vi "MH_T2 Read Acq QueueClassic.vi"() -> ()   [LabVIEW 2019]
uses:
  <userlib>/MultiHarp150/T2Lib/MH_T2QMessage.ctl
  <userlib>/MultiHarp150/T2Lib/MH_T2DeltaQMessage.ctl
panel:
  in  "Dbuffsize":i32=10
  out "Done":bool
  out "TotalRec":i32
  out "TotalTime":u32
  in  "stop":bool
  out "sortie d'erreur":errorcluster caption="ErrorOut"
  out "RollOver":bool
  in  "BufSze":i32=1000000
  in  "entrée d'erreur":errorcluster caption="ErrorIn"
  in  "WIndowW":i32
  in  "Save Data":bool
  in  "Correl Ch":u32=2
  in  "Base Ch":u32=1
  in  "refnum":refnum<file>
  out "DeltaT":u32[](array[numeric])
  out "nActual":i32[](array[numeric])
  out "En Attente":i32[](array[numeric])
  out "Tableau":u64[][](array[numeric])
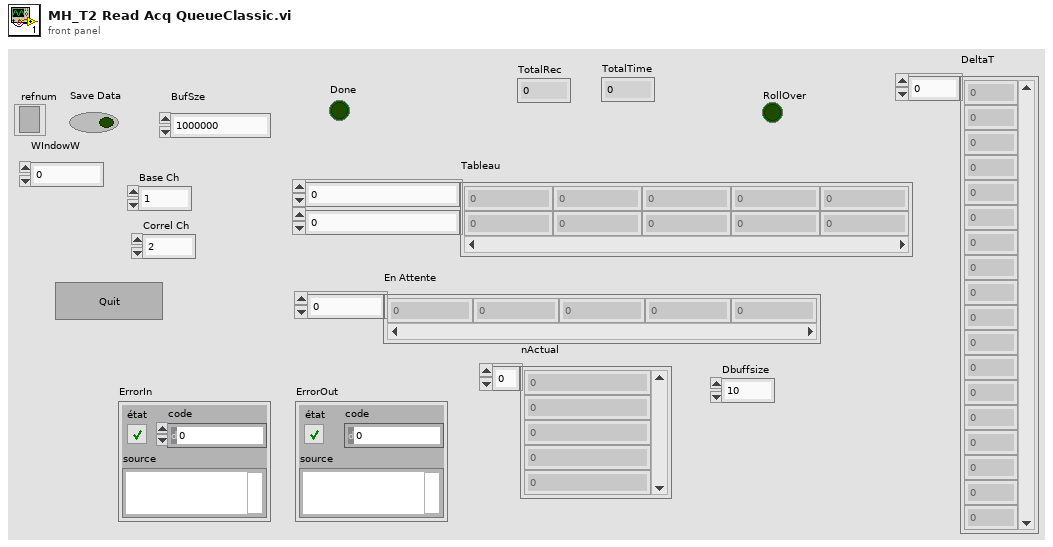
[diagram p1: front panel]
types:
  T1 = typedef "MH_T2DeltaQMessage.ctl" = cluster{"Message":string, "buffer":i32[], "Code":i32, "nactual":i32}
  T2 = typedef "MH_T2QMessage.ctl" = cluster{"Message":string, "buffer":u32[], "Code":i32, "nactual":i32}
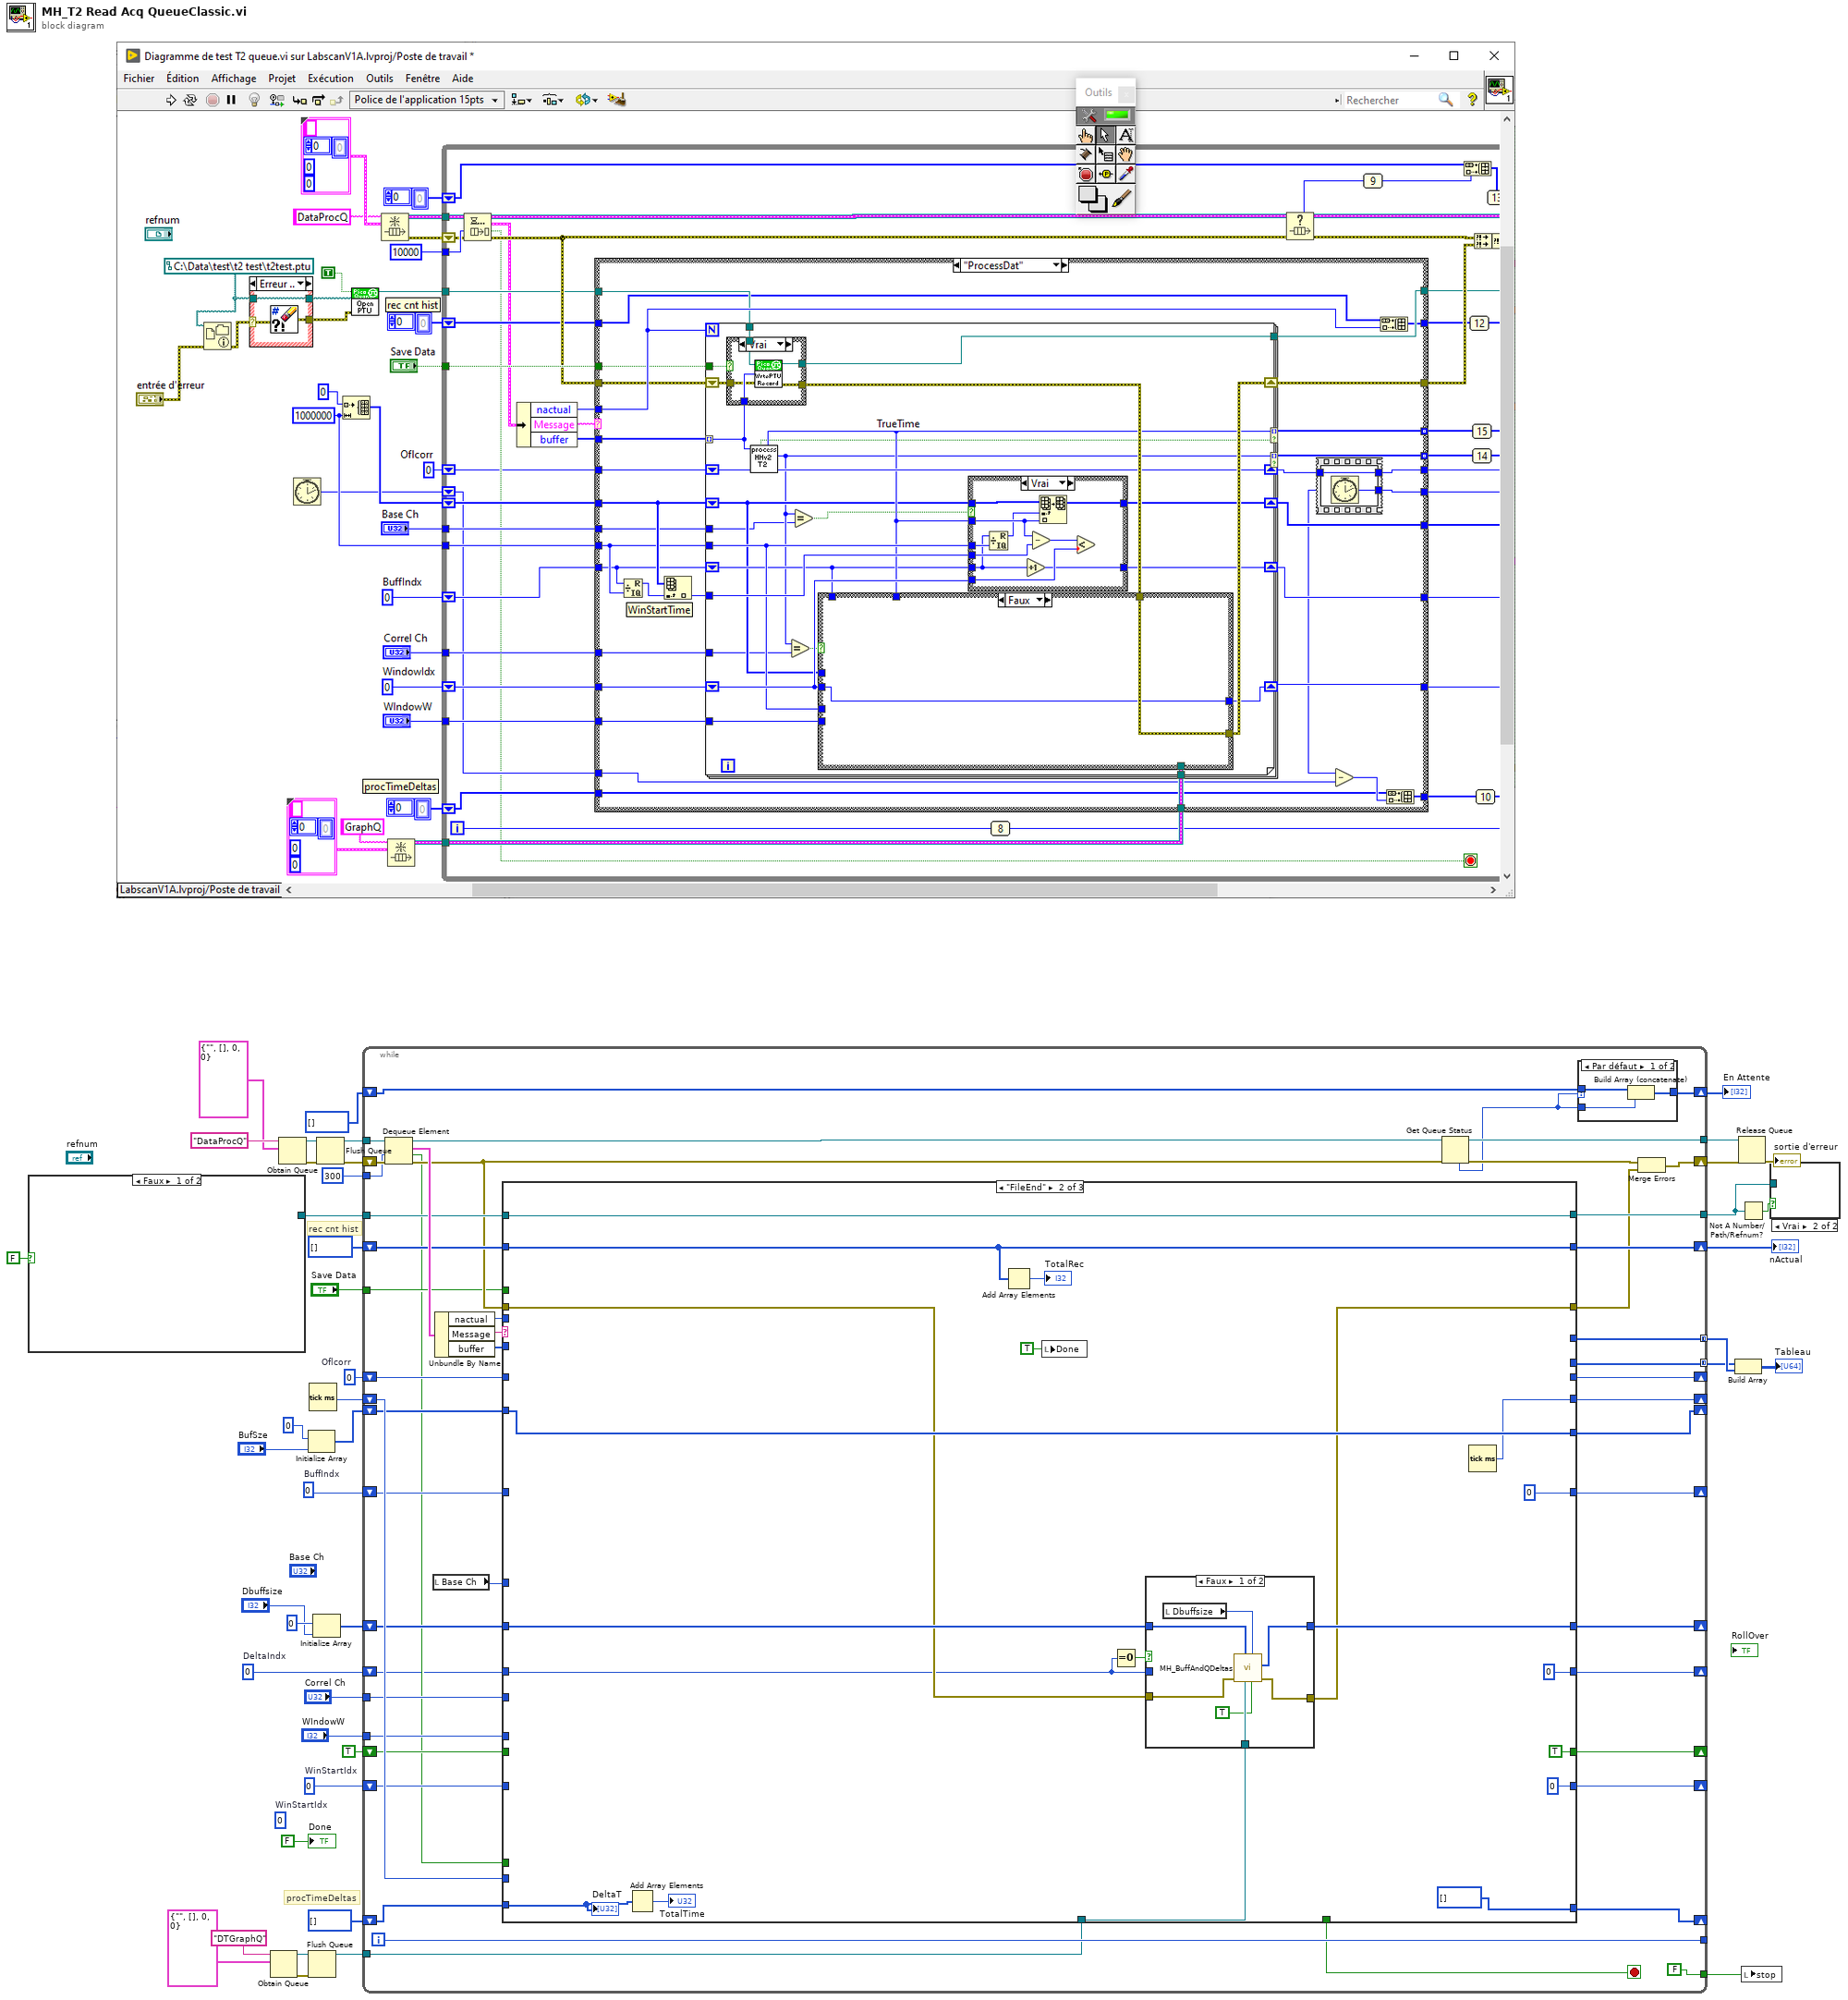
[diagram p0: block diagram]
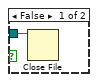
[diagram p2: hidden frame]
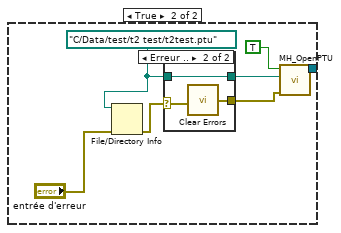
[diagram p3: hidden frame]
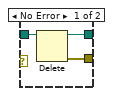
[diagram p4: hidden frame]
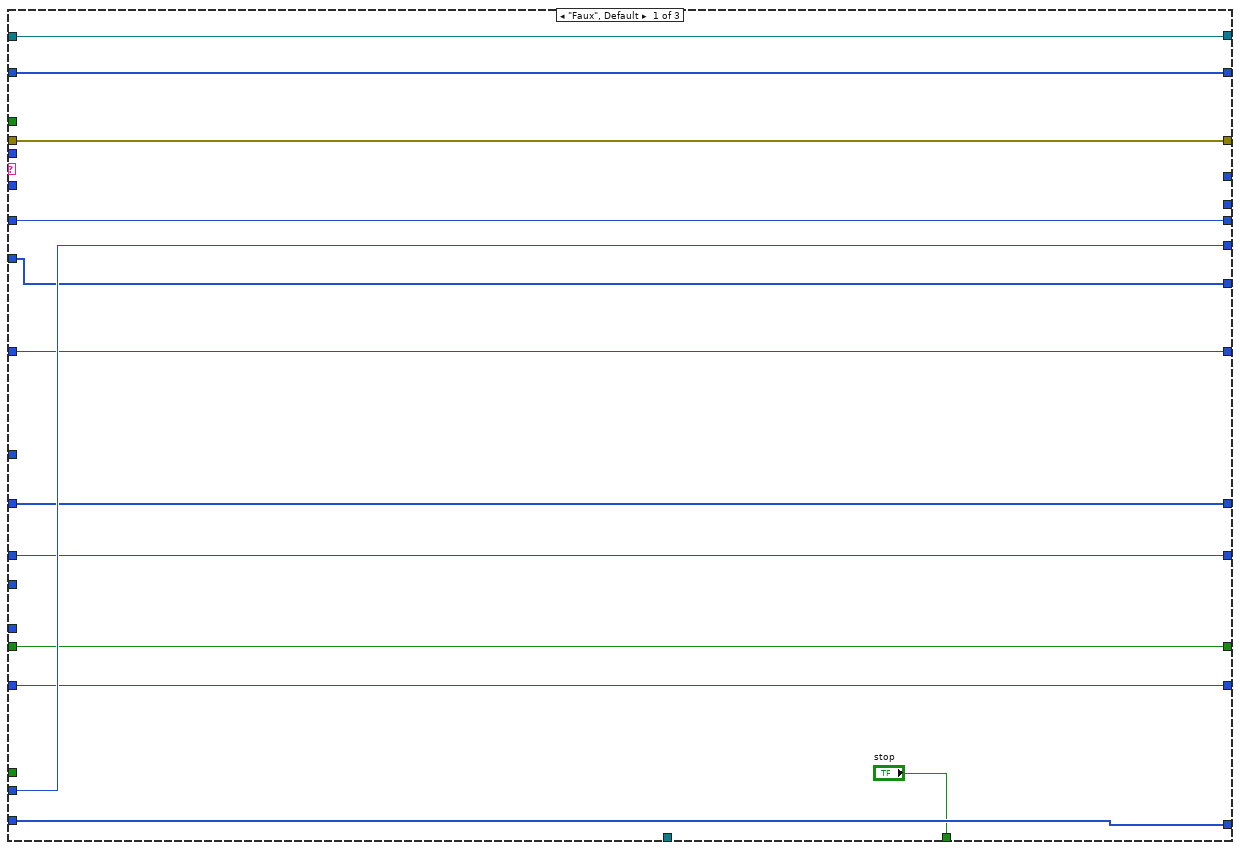
[diagram p6: hidden frame]
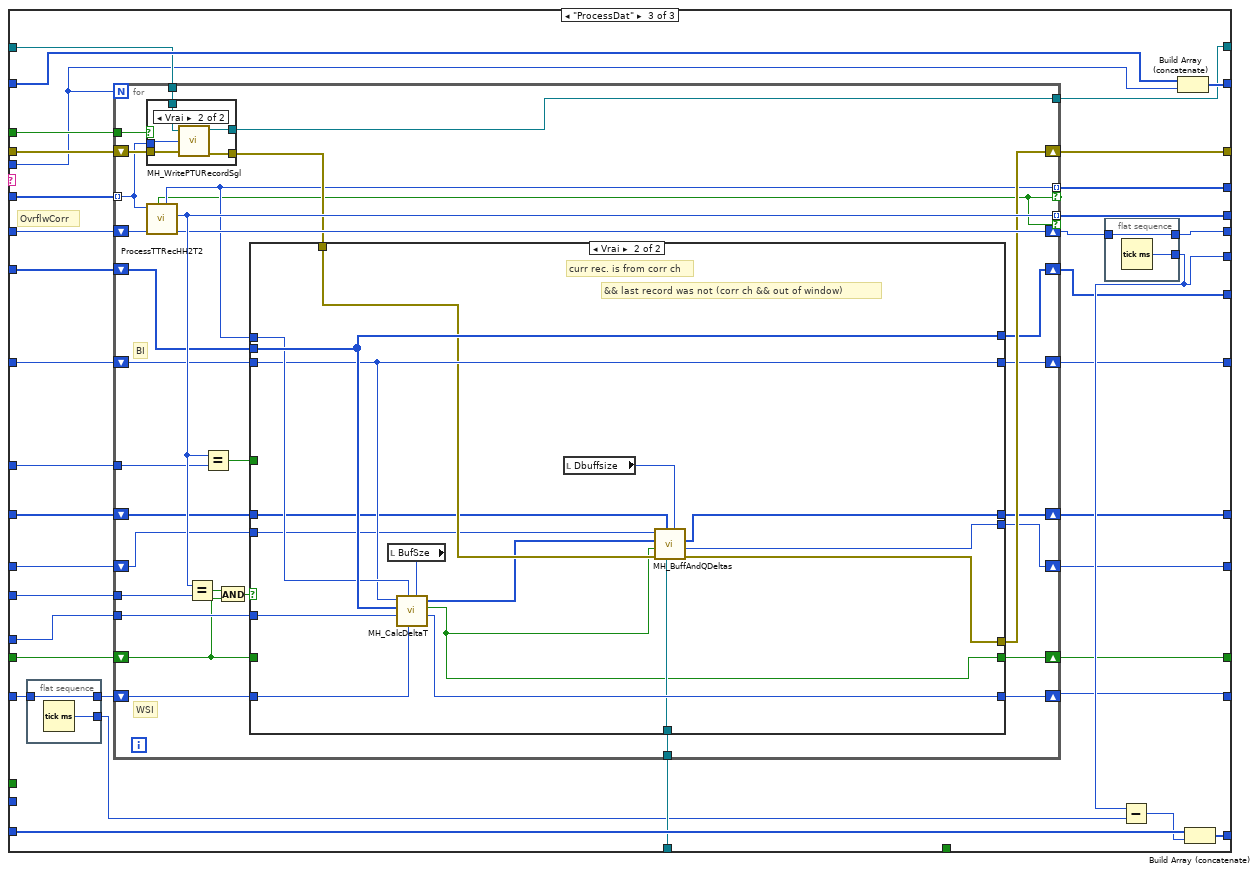
[diagram p8: hidden frame]
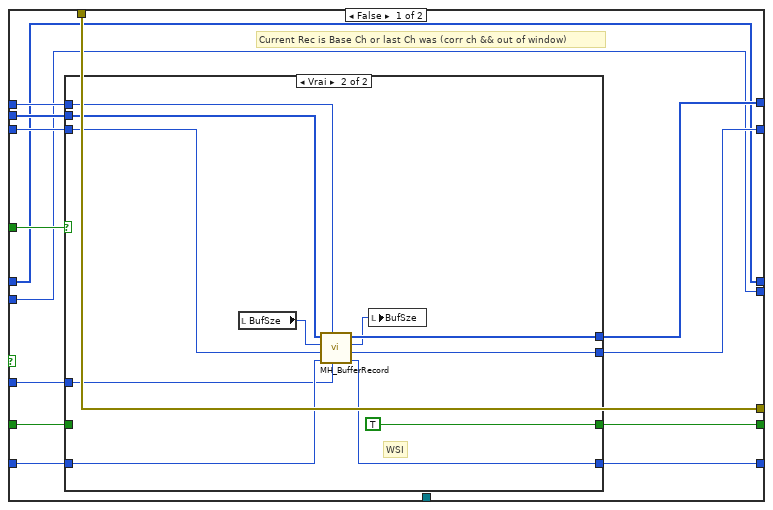
[diagram p10: hidden frame]
diagram:
  (unwired) 0  # WinStartIdx
  w3 = 0  # DeltaIndx
  w26 = 0  # WinStartIdx
  w14 = 0  # BuffIndx
  w42 = u64 0  # Oflcorr
  # "procTimeDeltas"
  # "rec cnt hist"
  n1 = case shown="Faux" FALSE {
    tunnel: [_ w50] -> w30
    frame False {
    }
    frame True {
      w47 = path "C:/Data/test/t2 test/t2test.ptu" ("chemin sélectionné")
      n2 = File/Directory Info(path=w47, error in="entrée d'erreur") -> (error out=w46:errorcluster)  [unwired: 6 out]
      n3 = case shown="Erreur .." w46 {
        selector: w46 -> [_ w56]
        tunnel: w47 -> [w54 w57]
        tunnel: [w53 w57] -> w49
        tunnel: [w52 w55] -> w48
        frame No Error {
          n4 = Delete(path (use dialog)=w54) -> (deleted path=w53:path, error out=w52:errorcluster)  [unwired: 4 in, 1 out]
        }
        frame Error {
          n5 = call <vilib>:"Clear Errors.vi"("error in (no error)"=w56) -> ("error out"=w55:errorcluster)  [unwired: 5 in, 1 out]
        }
      }
      n6 = call <userlib>:"MH_OpenPTU.vi"("ErrorIn"=w48, "chemin sélectionné"=w49, "WriteMode"=TRUE) -> ("refnum en sortie"=w50:refnum<file>)  [unwired: 6 in, 2 out]
    }
  }
  n7 = Obtain Queue(name (unnamed)="DTGraphQ" ("nom (aucun)"), element data type=T1 {"Message"="", "buffer"=[], "Code"=0, "nactual"=0} ("ClassQueue")) -> (queue out=w5:refnum<queue>, error out=w6:errorcluster)  [unwired: 3 in, 1 out]
  n8 = Obtain Queue(name (unnamed)="DataProcQ" ("nom (aucun)"), element data type=T2 {"Message"="", "buffer"=[], "Code"=0, "nactual"=0} ("ClassQueue")) -> (queue out=w11:refnum<queue>, error out=w8:errorcluster)  [unwired: 3 in, 1 out]
  n9 = Initialize Array(u64 0 ("truetime"), "BufSze") -> (w1:u64[])
  n10 = Flush Queue(queue=w5, error in (no error)=w6) -> (queue out=w16:refnum<queue>)  [unwired: 2 out]
  n11 = Tick Count (ms)() -> (millisecond timer value=w35:u32)
  n12 = Initialize Array(0 ("truetime"), "Dbuffsize") -> (w12:i32[])
  n13 = Flush Queue(queue=w11, error in (no error)=w8) -> (queue out=w10:refnum<queue>, error out=w9:errorcluster)  [unwired: 1 out]
  n14 = while {
    tunnel: w10 -> [w105]
    shift-right: [w83] -> w41
    shift-left: w9 -> [w106]
    shift-right: [w103] -> _
    shift-left: w42 -> [w104]
    tunnel: [w102] -> w38 mode=concatenating
    tunnel: [w99] -> _
    tunnel: [w95] -> w40
    tunnel: [w94] -> w37 mode=concatenating
    shift-right: [w92] -> _
    shift-left: w35 -> [w93]
    shift-right: [w90] -> _
    shift-left: u32[] [] ("DeltaT") -> [w91]
    shift-right: [w88] -> w32
    shift-left: i32[] [] ("DeltaT") -> [w89]
    shift-right: [w87] -> w39
    shift-left: i32[] [] ("DeltaT") -> [w86]
    tunnel: w30 -> [w85]
    tunnel: [w82] -> w19
    tunnel: "Save Data" -> [w81]
    shift-right: [w76] -> _
    shift-left: w1 -> [w80]
    shift-right: [w78] -> _
    shift-left: w14 -> [w79]
    tunnel: "Correl Ch" -> [w77]
    shift-right: [w72] -> _
    shift-left: w26 -> [w75]
    tunnel: "WIndowW" -> [w74]
    tunnel: 300 ("timeout en ms (-1)") -> [w73]
    tunnel: w16 -> [w70]
    shift-right: [w68] -> _
    shift-left: TRUE -> [w67]
    shift-right: [w65] -> _
    shift-left: w12 -> [w66]
    tunnel: [FALSE] -> w4
    shift-right: [w59] -> _
    shift-left: w3 -> [w60]
    i -> [w99]
    stop <- w63 stop-if-true
    n15 = Dequeue Element(queue=w105, timeout in ms (-1)=w73, error in (no error)=w106) -> (queue out=w97:refnum<queue>, element=w101:T2, timed out?=w64:bool, error out=w84:errorcluster)
    n16 = local read "Base Ch"() -> (w58:u32)
    n17 = Unbundle By Name(w101) -> ("nactual"=w71:i32, "Message"=w98:string, "buffer"=w100:u32[])
    n18 = case shown="\"FileEnd\"" w98 {
      tunnel: w104 -> [w123 _ w188]
      tunnel: [w123 _ w185] -> w103
      tunnel: [_ _ w187] -> w102
      tunnel: w100 -> [_ _ w178]
      tunnel: [_ _ w186] -> w94
      tunnel: w93 -> [w122 _ _]
      tunnel: [w121 u32[] [] ("DeltaT") w182] -> w90
      tunnel: [w122 w141 w179] -> w92
      tunnel: w91 -> [w121 w139 w184]
      tunnel: w89 -> [w120 w136 w181]
      tunnel: [w120 w136 w180] -> w88
      tunnel: w85 -> [w119 w143 w177]
      tunnel: w84 -> [w115 w127 w176]
      tunnel: [w119 w143 w175] -> w82
      tunnel: w81 -> [_ _ w174]
      tunnel: w80 -> [w117 w142 w163]
      tunnel: w79 -> [w118 _ w164]
      tunnel: [w118 0 ("BuffIndx") w172] -> w78
      tunnel: w77 -> [_ _ w173]
      tunnel: [w117 w142 w171] -> w76
      tunnel: w75 -> [w116 _ w157]
      tunnel: w74 -> [_ _ w170]
      tunnel: [w116 0 ("WinStartIdx") w168] -> w72
      tunnel: w71 -> [_ _ w167]
      tunnel: w70 -> [_ w126 w166]
      tunnel: [w115 w128 w165] -> w69
      tunnel: [w114 TRUE w162] -> w68
      tunnel: w67 -> [w114 _ w161]
      tunnel: w66 -> [w113 w130 w160]
      tunnel: [w113 w129 w159] -> w65
      tunnel: w64 -> [_ _ _]
      tunnel: ["stop" _ _] -> w63
      tunnel: w60 -> [w111 w125 w155]
      tunnel: [w111 0 w154] -> w59
      tunnel: w58 -> [_ _ w153]
      frame "Faux", Default {
      }
      frame "FileEnd" {
        n19 = Add Array Elements(numeric array=w139) -> (sum=→"TotalTime":u32)
        n20 = Add Array Elements(numeric array=w136) -> (sum=→"TotalRec":i32)
        n21 = local write "Done"(TRUE ("Done")) -> ()
        n22 = Equal To 0?(x=w125) -> (x = 0?=w124:bool)
        n23 = case shown="Faux" w124 {
          tunnel: w130 -> [w146 w152]
          tunnel: [w150 w152] -> w129
          tunnel: [w149 w151] -> w128
          tunnel: w127 -> [w148 w151]
          tunnel: w125 -> [_ _]
          tunnel: w126 -> [w147 _]
          frame False {
            n24 = local read "Dbuffsize"() -> (w145:i32)
            n25 = call <userlib>:"MH_BuffAndQDeltas.vi"("Force Write"=TRUE ("NewDelta"), "DBuffSize"=w145, "queue out"=w147, "DeltasBuffer"=w146, "erroIn"=w148) -> ("error out"=w149:errorcluster, "DeltasBufferOut"=w150:i32[])  [unwired: 4 in, 1 out]
          }
          frame True {
          }
        }
        n26 = Tick Count (ms)() -> (millisecond timer value=w141:u32)
        "DeltaT" <- w139
      }
      frame "ProcessDat" {
        # "OvrflwCorr"
        n27 = flat-sequence {
          tunnel: [w190] -> w156
          tunnel: w157 -> [w190]
          tunnel: [w189] -> w158
          frame #0 {
            n28 = Tick Count (ms)() -> (millisecond timer value=w189:u32)
          }
        }
        n29 = for {
          N: w167 -> [_]
          tunnel: [w205] -> w187 mode=indexing if=w196
          tunnel: w178 -> [w219] mode=indexing
          tunnel: [w217] -> w186 mode=indexing if=w196
          tunnel: w177 -> [w222]
          tunnel: [w220] -> w175
          tunnel: w174 -> [w218]
          shift-right: [w202] -> w171
          shift-left: w163 -> [w206]
          shift-right: [w203] -> w172
          shift-left: w164 -> [w204]
          tunnel: w173 -> [w215]
          tunnel: w170 -> [w214]
          shift-right: [w213] -> w169
          shift-left: w188 -> [w223]
          shift-right: [w212] -> w168
          shift-left: w156 -> [w208]
          shift-right: [w209] -> w165
          shift-left: w176 -> [w221]
          tunnel: w166 -> [w211]
          shift-right: [w201] -> w162
          shift-left: w161 -> [w199]
          shift-right: [w197] -> w159
          shift-left: w160 -> [w198]
          shift-right: [w194] -> w154
          shift-left: w155 -> [w195]
          tunnel: w153 -> [w193]
          # "BI"
          # "WSI"
          n30 = case shown="Vrai" w218 {
            tunnel: w222 -> [w224 w230]
            tunnel: w221 -> [w225 w229]
            tunnel: [w224 w228] -> w220
            tunnel: [w225 w227] -> w210
            tunnel: w219 -> [_ w226]
            frame False {
            }
            frame True {
              n31 = call <userlib>:"MH_WritePTURecordSgl.vi"("refnum"=w230, "TTTR Records"=w226, "error in"=w229) -> ("refnum en sortie"=w228:refnum<file>, "error out"=w227:errorcluster)  [unwired: 6 in]
            }
          }
          n32 = call <userlib>:"ProcessTTRecHH2T2.vi"("oflcorr_in"=w223, "rawbits"=w219) -> ("oflcorr_out"=w213:u64, "channel"=w217:u32, "truetime"=w205:u64, "is_photon"=w196:bool)  [unwired: 4 in, 2 out]
          n33 = Equal?(x=w217, y=w215) -> (x = y?=w216:bool)
          n34 = Equal?(x=w217, y=w193) -> (x = y?=w207:bool)
          n35 = And(x=w216, y=w199) -> (x .and. y?=w200:bool)
          n36 = case shown="Vrai" w200 {
            tunnel: w206 -> [w242 w276]
            tunnel: w208 -> [w238 w271]
            tunnel: w204 -> [w240 w273]
            tunnel: w214 -> [w236 w272]
            tunnel: [w235 w270] -> w212
            tunnel: w211 -> [_ w266]
            tunnel: w210 -> [w244 w269]
            tunnel: [w244 w265] -> w209
            tunnel: w207 -> [w241 _]
            tunnel: w205 -> [w237 w275]
            tunnel: [w239 w273] -> w203
            tunnel: [w243 w276] -> w202
            tunnel: [w234 w263] -> w201
            tunnel: w199 -> [w233 _]
            tunnel: w198 -> [w232 w262]
            tunnel: [w232 w268] -> w197
            tunnel: w195 -> [w231 w261]
            tunnel: [w231 w267] -> w194
            frame False {
              # "Current Rec is Base Ch or last Ch was (corr ch && out of window)"
              n37 = case shown="Vrai" w241 {
                tunnel: w242 -> [w247 w251]
                tunnel: w237 -> [_ w250]
                tunnel: w240 -> [w248 w254]
                tunnel: [w248 w258] -> w239
                tunnel: [w247 w257] -> w243
                tunnel: w238 -> [w246 w255]
                tunnel: w236 -> [_ w249]
                tunnel: [w246 w256] -> w235
                tunnel: [w245 TRUE] -> w234
                tunnel: w233 -> [w245 _]
                frame False {
                  # "could be sync or non-relevant channel"
                }
                frame True {
                  # "WSI"
                  n38 = local read "BufSze"() -> (w253:i32)
                  n39 = call <userlib>:"MH_BufferRecord.vi"("WindowWidth"=w249, "truetime"=w250, "WinIndex"=w255, "Buffindex"=w254, "Buffsize"=w253, "Buffer"=w251) -> ("WinIndexOut"=w256:i32, "BuffIndexOut"=w258:i32, "NewBuffsize"=w252:i32, "tableau (n rotations)"=w257:u64[])  [unwired: 2 in]
                  n40 = local write "BufSze"(w252) -> ()
                }
              }
            }
            frame True {
              # "&& last record was not (corr ch && out of window)"
              # "curr rec. is from corr ch"
              n41 = local read "BufSze"() -> (w274:i32)
              n42 = call <userlib>:"MH_CalcDeltaT.vi"("Buffsize"=w274, "WinIndex"=w271, "TrueTime"=w275, "WIndowW"=w272, "Data In"=w276, "Buffindex"=w273) -> ("WinIndexOut"=w270:i32, "NewDelta"=w263:bool, "DeltaT Out"=w260:i32[])  [unwired: 3 in]
              n43 = local read "Dbuffsize"() -> (w264:i32)
              n44 = call <userlib>:"MH_BuffAndQDeltas.vi"("DBuffSize"=w264, "queue out"=w266, "DeltasBuffer"=w262, "erroIn"=w269, "NewDelta"=w263, "Deltas In"=w260, "Deltaindex"=w261) -> ("error out"=w265:errorcluster, "DeltaIndexOut"=w267:i32, "DeltasBufferOut"=w268:i32[])  [unwired: 2 in]
            }
          }
        }
        n45 = flat-sequence {
          tunnel: [w192] -> w185
          tunnel: w169 -> [w192]
          tunnel: [w191] -> w179
          frame #0 {
            n46 = Tick Count (ms)() -> (millisecond timer value=w191:u32)
          }
        }
        n47 = Subtract(x=w179, y=w158) -> (x-y=w183:u32)
        n48 = Build Array (concatenate)(w181, w167) -> (w180:i32[])
        n49 = Build Array (concatenate)(w184, w183) -> (w182:u32[])
      }
    }
    n50 = Get Queue Status(queue=w97, error in (no error)=w84) -> (queue out=w95:refnum<queue>, error out=w96:errorcluster, # elements in queue=w61:i32)  [unwired: 1 in, 5 out]
    n51 = case shown="Par défaut" w61 {
      tunnel: w61 -> [w109 _]
      tunnel: [w108 w110] -> w87
      tunnel: w86 -> [w107 w110]
      frame Default {
        n52 = Build Array (concatenate)(w107, w109) -> (w108:i32[])
      }
      frame 0 {
      }
    }
    n53 = Merge Errors(w96, w69) -> (w83:errorcluster)
  }
  "En Attente" <- w39
  "nActual" <- w32
  n54 = Build Array(w37, w38) -> (→"Tableau":u64[][])
  n55 = Release Queue(queue=w40, error in (no error)=w41) -> (error out=→"sortie d'erreur":errorcluster)  [unwired: 1 in, 2 out]
  n56 = Not A Number/Path/Refnum?(number/path/refnum=w19) -> (NaN/Path/Refnum?=w18:bool)
  n57 = local write "stop"(w4) -> ()
  n58 = case shown="Vrai" w18 {
    tunnel: w19 -> [w277 _]
    frame False {
      n59 = Close File(refnum=w277) -> ()  [unwired: 1 in, 2 out]
    }
    frame True {
    }
  }
  "Done" <- FALSE
